vi "HQ Main.vi"() -> ()   [LabVIEW 2015]
uses:
  Type Defs/Air Bearing.ctl
panel:
  in  "Test Run Config":bool
  in  "Stop Pod":bool
  in  "Close Down HQ":bool
  in  "History":bool
  in  "Filght Run":bool
  in  "Pod Loading":bool
  in  "Phase":T1(tab)
  out "Flight Phase":T2
  in  "Initiate Launch":bool
  out "Awaiting Launch Command":bool
  out "Final Check":bool
  out "Power":T3 {"Battery (Secondary)" scale=0.0..100.0; "Battery (Primary)" scale=0.0..100.0; "System Power Consumption" scale=0.0..10.0}
  out "Thermal":T4 {"T 6" scale=0.0..150.0; "T 5" scale=0.0..150.0; "T 4" scale=0.0..150.0; "T 3" scale=0.0..150.0; "T 2" scale=0.0..150.0; "T 1" scale=0.0..150.0}
  in  "Intertial Measurement Unit":T5={"Accelerometer"={"X"=3.2323232323232323, "Y"=3.2323232323232323, "Z"=3.2323232323232323}, "Gyroscope"={"P"=3.2323232323232323, "Y"=3.2323232323232323, "R"=3.2323232323232323}, "Magnetometer"={"X"=3.2323232323232323, "Y"=3.2323232323232323, "Z"=3.2323232323232323}} {"Magnetometer"."Z" scale=0.0..10.0; "Magnetometer"."Y" scale=0.0..10.0; "Magnetometer"."X" scale=0.0..10.0; "Gyroscope"."R" scale=0.0..10.0; "Gyroscope"."Y" scale=0.0..10.0; "Gyroscope"."P" scale=0.0..10.0; "Accelerometer"."Z" scale=0.0..10.0; "Accelerometer"."Y" scale=0.0..10.0; "Accelerometer"."X" scale=0.0..10.0}
  out "Progress Log":string
  in  "Detailed Telemetry":T6(tab)
  out "Temperature":dbl[](graph)
  out "Pusher Engaged":bool
  out "Air Bearings":T8={"Air Bearing 1"={"Pressurized"=FALSE, "Air Gap (mm)"=8.775510204081632, "Air Left"=0.0}, "Air Bearing 2"={"Pressurized"=FALSE, "Air Gap (mm)"=8.775510204081632, "Air Left"=0.0}, "Air Bearing 3"={"Pressurized"=FALSE, "Air Gap (mm)"=8.775510204081632, "Air Left"=0.0}, "Air Bearing 4"={"Pressurized"=FALSE, "Air Gap (mm)"=8.775510204081632, "Air Left"=0.0}} {"Air Bearing 4"."Air Left" format="%#_g%"; "Air Bearing 4"."Air Gap (mm)" scale=0.0..20.0; "Air Bearing 3"."Air Left" format="%#_g%"; "Air Bearing 3"."Air Gap (mm)" scale=0.0..20.0; "Air Bearing 2"."Air Left" format="%#_g%"; "Air Bearing 2"."Air Gap (mm)" scale=0.0..20.0; "Air Bearing 1"."Air Left" format="%#_g%"; "Air Bearing 1"."Air Gap (mm)" scale=0.0..20.0}
  out "Brakes (Magnetic)":bool
  out "Brakes (Friction)":bool
  out "Speed":dbl[](graph)
  out "Status":string
  out "Ready To Launch!":bool
  in  "Track Position":dbl(slide) scale=0.0..5000.0
  # "A, B, C, D\nPower-on & Diagnostics\nComms Check\n  Active\n  Latency\n  Bandwidth\nLevitation\nCalibration"
  # "Last Run\nRun Replay"
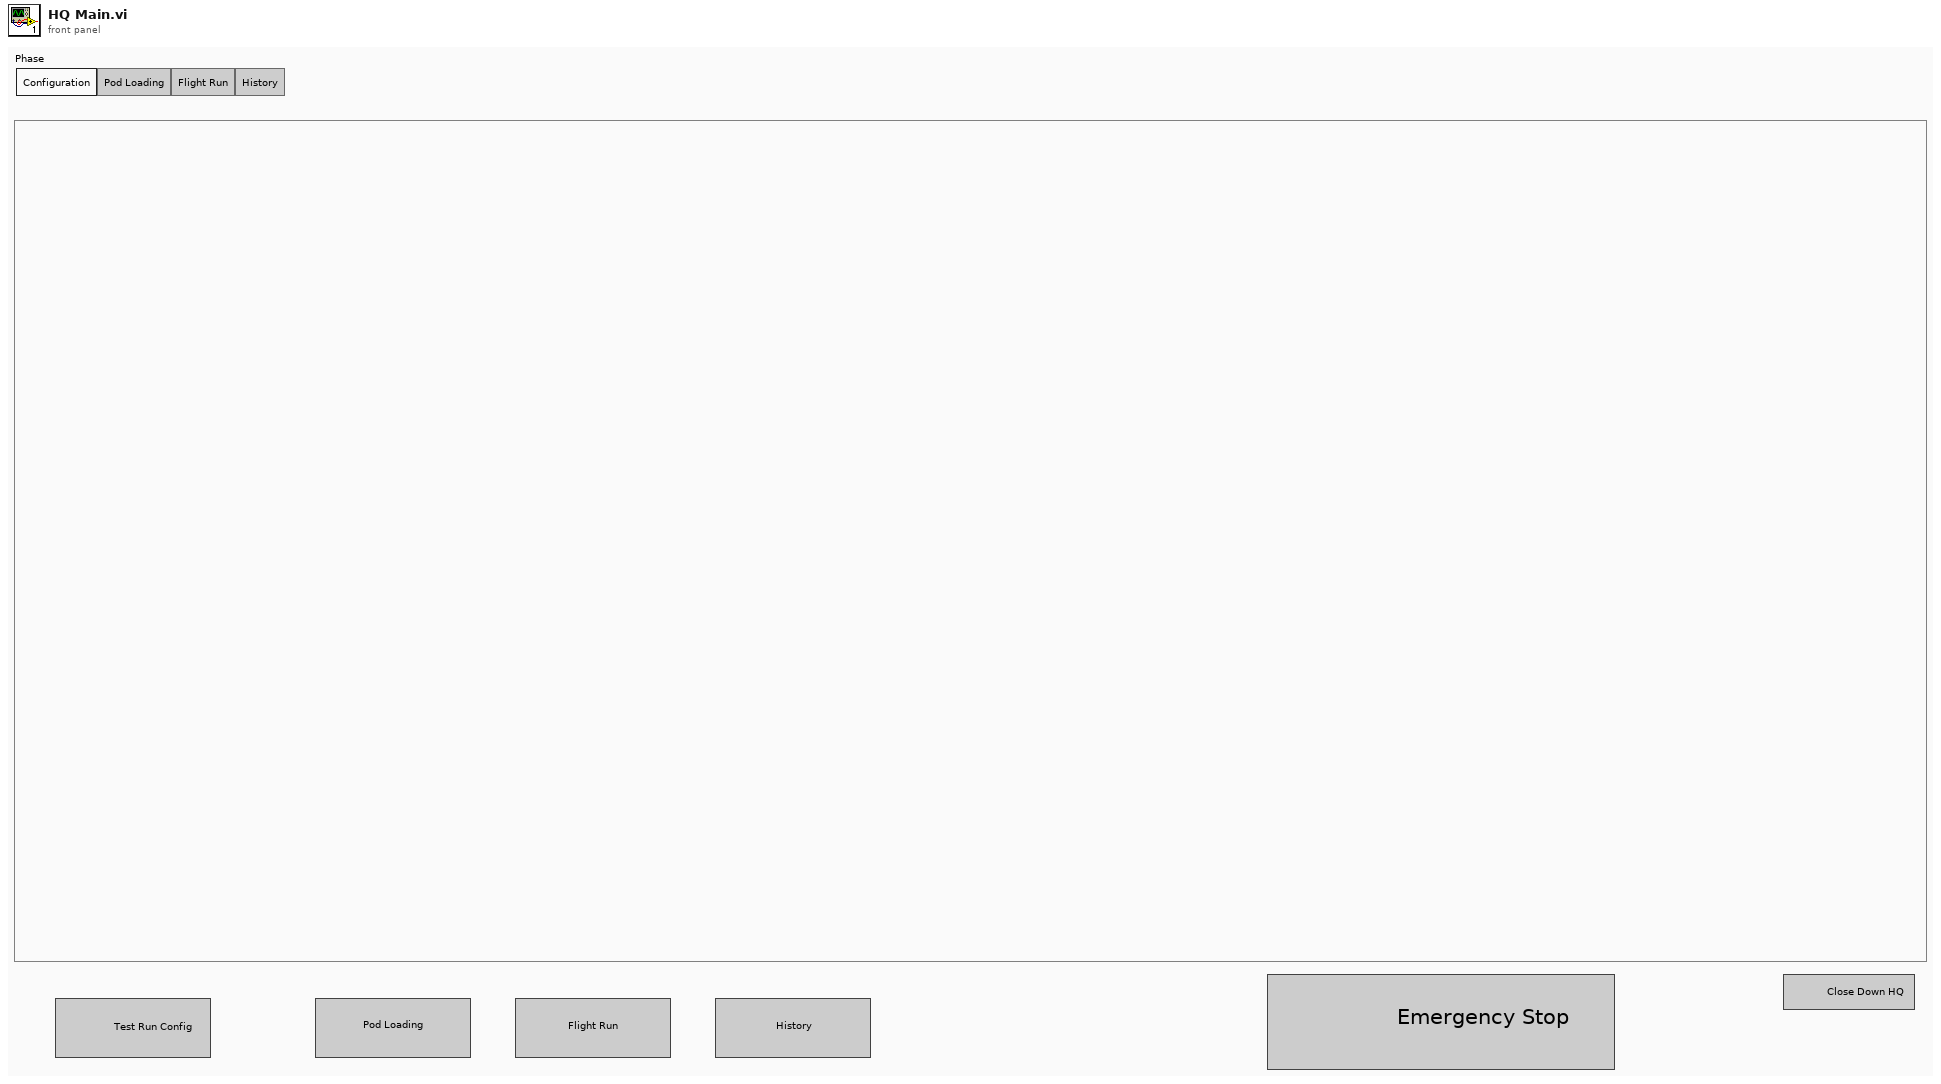
[diagram p1: front panel]
types:
  T1 = enum32{"Configuration", "Pod Loading", "Flight Run", "History"}
  T2 = cluster{"Acceleration":bool, "Coast":bool, "Deceleration":bool, "Stopped":bool}
  T3 = cluster{"System Power Consumption":dbl, "Battery (Primary)":u8, "Battery (Secondary)":u8}
  T4 = cluster{"T 1":dbl, "T 2":dbl, "T 3":dbl, "T 4":dbl, "T 5":dbl, "T 6":dbl}
  T5 = cluster{"Accelerometer":cluster{"X":dbl, "Y":dbl, "Z":dbl}, "Gyroscope":cluster{"P":dbl, "Y":dbl, "R":dbl}, "Magnetometer":cluster{"X":dbl, "Y":dbl, "Z":dbl}}
  T6 = enum32{"Thermal", "Power Consumption", "Accelerometer & Gyroscope", "Pressure & Levitation"}
  T7 = typedef "Air Bearing.ctl" = cluster{"Pressurized":bool, "Air Gap (mm)":dbl, "Air Left":dbl}
  T8 = cluster{"Air Bearing 1":T7, "Air Bearing 2":T7, "Air Bearing 3":T7, "Air Bearing 4":T7}
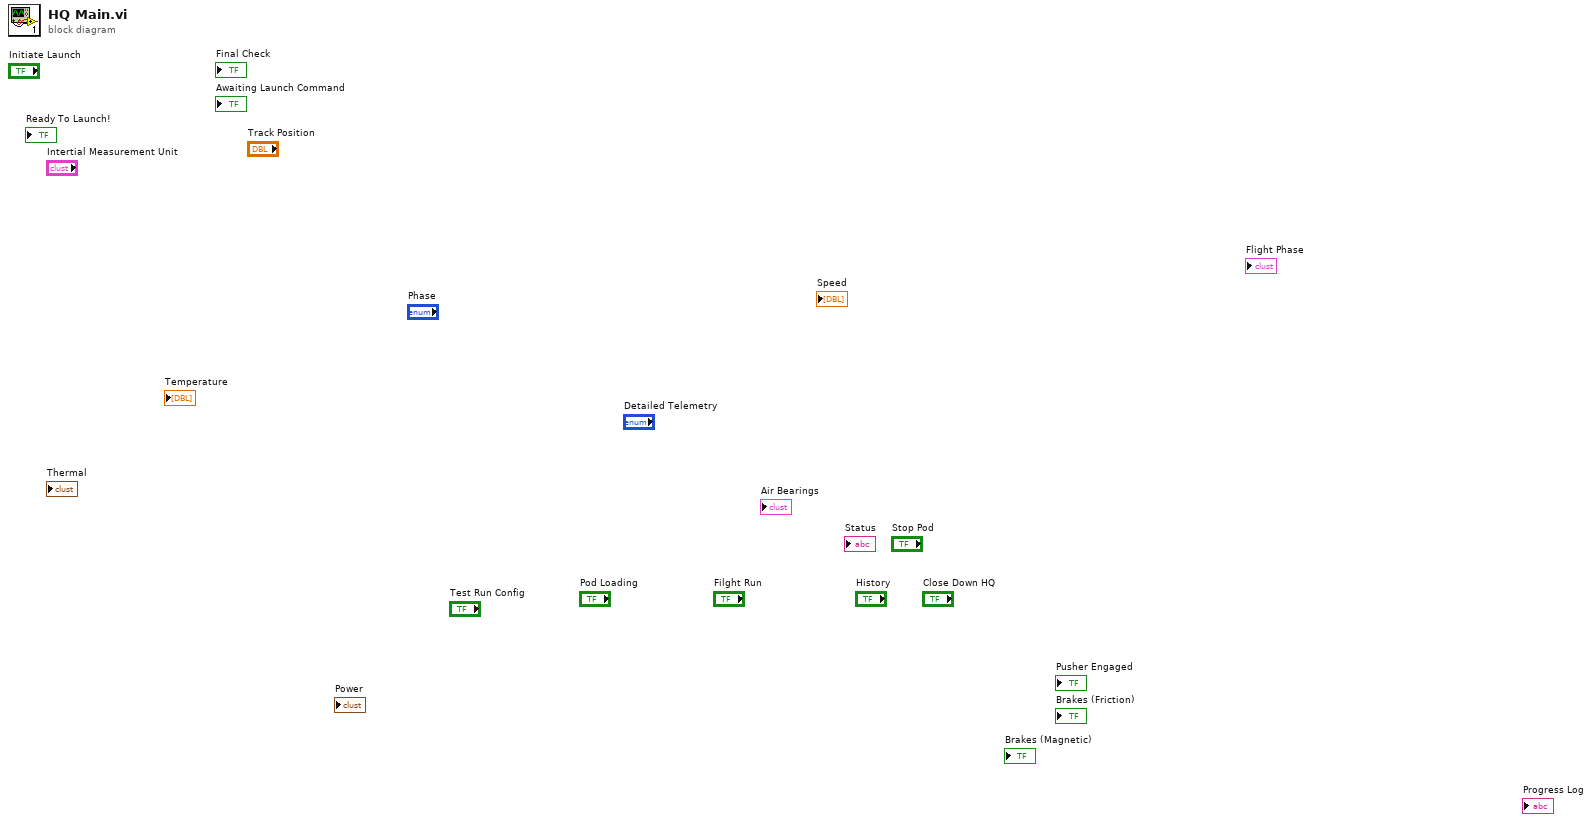
[diagram p0: block diagram]
diagram:
